vi "RealTimeMain.vi"(9 "For Reference (frames)":i32=1 min=1, 11 "Motion Data":T2(array[cluster])) -> (3 "Array":dbl[][](array[numeric]))   [LabVIEW 2014]
uses:
  GlobalVars.vi
panel:
  out "Averaging 2":bool
  in  "Col Shift Element":dbl[](array[numeric])
  in  "Vert SF":dbl[](array[numeric])
  in  "Row Shift Element":dbl[](array[numeric])
  in  "Horiz SF":dbl[](array[numeric])
  in  "Reference Frame":dbl[][][](array[numeric])
  in  "Header":T1
  in  "Ref Avg Count":i32
  in  "Alarm Structure":enum32{"Alarm", "Averaging"}(tab)=enum."Averaging"
  in  "Averaging":bool
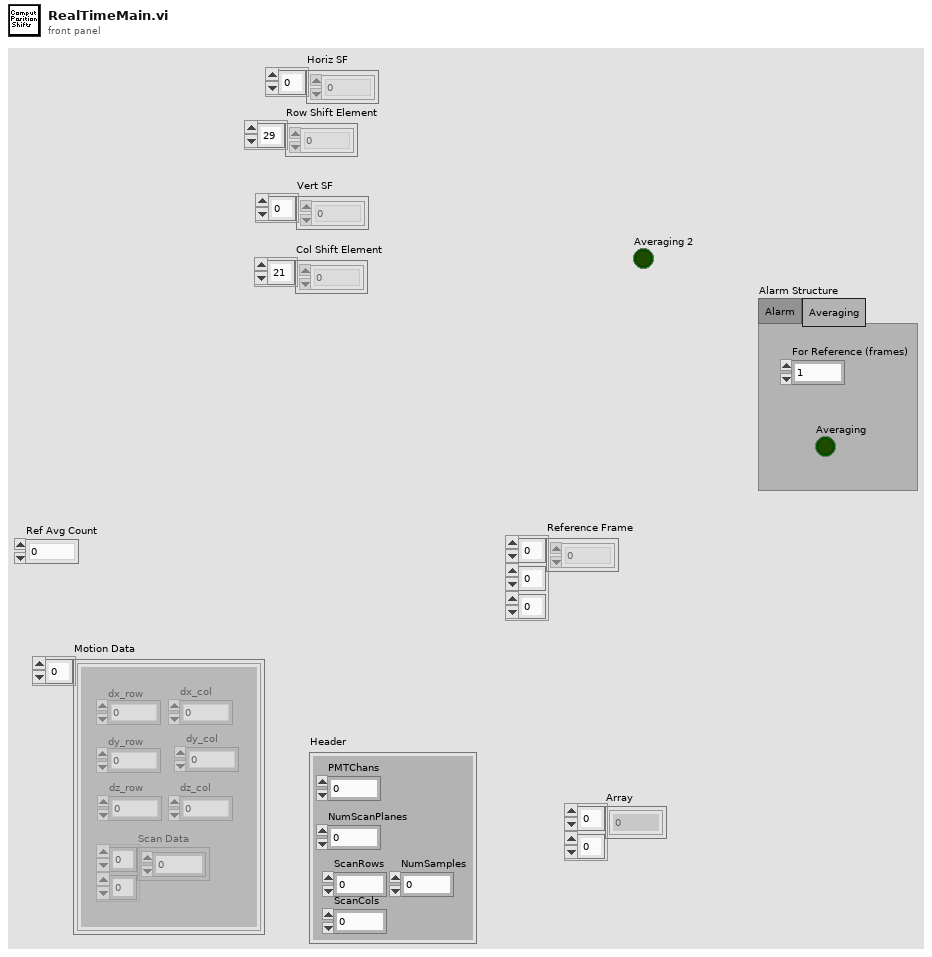
[diagram p1: front panel]
types:
  T1 = cluster{"PMTChans":i32, "NumScanPlanes":i32, "ScanRows":i32, "ScanCols":i32, "NumSamples":i32}
  T2 = cluster{"Scan Data":i32[][], "dx_row":dbl, "dy_row":dbl, "dz_row":dbl, "dx_col":dbl, "dy_col":dbl, "dz_col":dbl}[]
  T3 = cluster{"Scan Data":i32[][], "dx_row":dbl, "dy_row":dbl, "dz_row":dbl, "dx_col":dbl, "dy_col":dbl, "dz_col":dbl}
  T4 = cluster{"dx_row":dbl, "dy_row":dbl, "dz_row":dbl, "dx_col":dbl, "dy_col":dbl, "dz_col":dbl}
  T5 = cluster{"X1":dbl[], "Y1":dbl[], "Z1":dbl[], "X2":dbl[], "Y2":dbl[], "Z2":dbl[]}
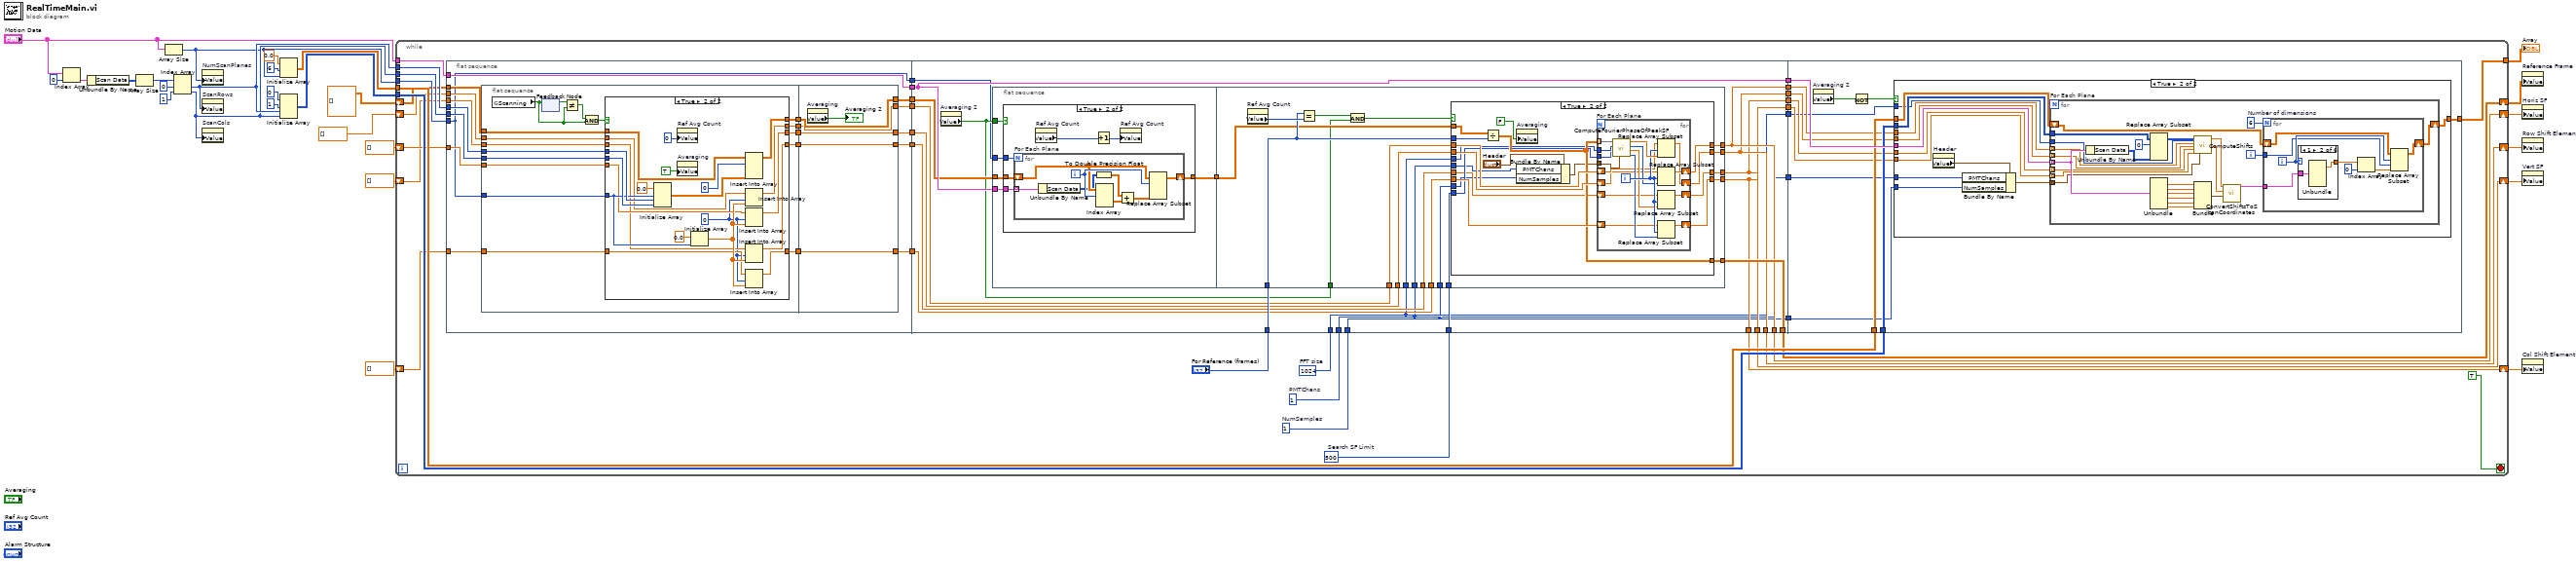
[diagram p0: block diagram]
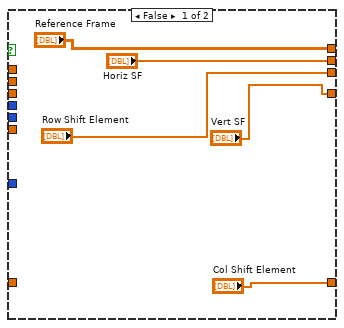
[diagram p2: hidden frame]
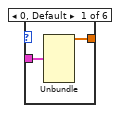
[diagram p6: hidden frame]
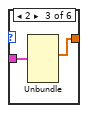
[diagram p7: hidden frame]
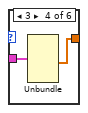
[diagram p8: hidden frame]
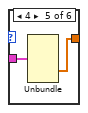
[diagram p9: hidden frame]
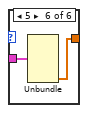
[diagram p10: hidden frame]
diagram:
  n1 = Index Array(array="Motion Data", index=0) -> (element=w26:T3)
  n2 = Unbundle By Name(w26) -> ("Scan Data"=w25:i32[][])
  n3 = Array Size(array=w25) -> (size(s)=w24:i32[])
  n4 = Array Size(array="Motion Data") -> (size(s)=w14:i32)
  n5 = Index Array(array=w24, index #1=0 ("index"), index #2=1 ("index")) -> (element #1=w17:i32, element #2=w16:i32)
  n6 = property on="NumScanPlanes" class="DigNum (strict)"("Value"=w14) -> ()  [unwired: 2 in, 2 out]
  n7 = property on="ScanRows" class="DigNum (strict)"("Value"=w17) -> ()  [unwired: 2 in, 2 out]
  n8 = property on="ScanCols" class="DigNum (strict)"("Value"=w16) -> ()  [unwired: 2 in, 2 out]
  n9 = Initialize Array(0.0 ("element"), 6 ("dimension size"), w14) -> (w12:dbl[][])
  n10 = Initialize Array(0 ("element"), 1 ("dimension size"), w17, w16) -> (w18:i32[][][])
  n11 = while {
    tunnel: "Motion Data" -> [w54]
    tunnel: w18 -> [w52]
    tunnel: w17 -> [w51]
    tunnel: w16 -> [w50]
    tunnel: w14 -> [w49]
    tunnel: w12 -> [w48]
    shift-right: [w42] -> w11
    shift-left: dbl[][][] [] -> [w35]
    tunnel: [w43] -> w6
    shift-right: [w41] -> w10
    shift-left: dbl[] [] -> [w47]
    shift-right: [w40] -> w9
    shift-left: dbl[] [] -> [w46]
    shift-right: [w39] -> w8
    shift-left: dbl[] [] -> [w45]
    shift-right: [w38] -> w7
    shift-left: dbl[] [] -> [w44]
    stop <- TRUE stop-if-true
    w30 = 1  # NumSamples
    w31 = 1  # PMTChans
    w34 = 500  # Search SF Limit
    w33 = 1024  # FFT size
    n12 = flat-sequence {
      tunnel: w54 -> [w84]
      tunnel: [w84] -> w65
      tunnel: w49 -> [w66]
      tunnel: w51 -> [w83]
      tunnel: w50 -> [w67]
      tunnel: w35 -> [w82]
      tunnel: [w81] -> w64
      tunnel: w47 -> [w80]
      tunnel: w46 -> [w79]
      tunnel: w45 -> [w78]
      tunnel: w44 -> [w77]
      tunnel: [w76] -> w63
      tunnel: [w75] -> w62
      tunnel: [w74] -> w61
      tunnel: [w73] -> w60
      tunnel: [w66] -> w37
      tunnel: w65 -> [w150]
      tunnel: "For Reference (frames)" -> [w152]
      tunnel: [w150] -> w59
      tunnel: w64 -> [w149]
      tunnel: w63 -> [w148]
      tunnel: w62 -> [w147]
      tunnel: w61 -> [w146]
      tunnel: w60 -> [w145]
      tunnel: [w142] -> w58
      tunnel: [w141] -> w57
      tunnel: [w140] -> w56
      tunnel: [w139] -> w55
      tunnel: [w143] -> w42
      tunnel: [w142] -> w41
      tunnel: [w141] -> w40
      tunnel: [w140] -> w39
      tunnel: [w139] -> w38
      tunnel: w37 -> [w138]
      tunnel: w33 -> [w136]
      tunnel: w34 -> [w137]
      tunnel: [w136] -> w32
      tunnel: w31 -> [w134]
      tunnel: w30 -> [w135]
      tunnel: [w135] -> w29
      tunnel: [w134] -> w28
      tunnel: w59 -> [w244]
      tunnel: w52 -> [w243]
      tunnel: w48 -> [w242]
      tunnel: w58 -> [w241]
      tunnel: w57 -> [w240]
      tunnel: w56 -> [w239]
      tunnel: w55 -> [w238]
      tunnel: [w237] -> w43
      tunnel: w32 -> [w234]
      tunnel: w29 -> [w233]
      tunnel: w28 -> [w232]
      frame #0 {
        n13 = flat-sequence {
          tunnel: w66 -> [w101]
          tunnel: w83 -> [w100]
          tunnel: w67 -> [w99]
          tunnel: w82 -> [w98]
          tunnel: w80 -> [w96]
          tunnel: w79 -> [w95]
          tunnel: w78 -> [w94]
          tunnel: w77 -> [w93]
          tunnel: [w97] -> w72
          tunnel: [w92] -> w71
          tunnel: [w91] -> w70
          tunnel: [w90] -> w69
          tunnel: [w89] -> w68
          tunnel: [w129] -> w73
          tunnel: [w130] -> w74
          tunnel: [w131] -> w75
          tunnel: [w132] -> w76
          tunnel: [w133] -> w81
          tunnel: w72 -> [w133]
          tunnel: w71 -> [w132]
          tunnel: w70 -> [w131]
          tunnel: w69 -> [w130]
          tunnel: w68 -> [w129]
          frame #0 {
            n14 = global read "GlobalVars.vi" "Scanning"() -> (w86:bool)
            n15 = feedback-in #1(w86) -> ()
            n16 = feedback #1() -> (w88:bool)  [unwired: 1 in]
            n17 = Not Equal?(x=w88, y=w86) -> (x != y?=w87:bool)
            n18 = And(x=w87, y=w86) -> (x .and. y?=w85:bool)
            n19 = case shown="True" w85 {
              tunnel: w101 -> [_ w119]
              tunnel: w100 -> [_ w126]
              tunnel: w99 -> [_ w125]
              tunnel: w98 -> [_ w124]
              tunnel: ["Reference Frame" w122] -> w97
              tunnel: w96 -> [_ w118]
              tunnel: w95 -> [_ w116]
              tunnel: w94 -> [_ w115]
              tunnel: w93 -> [_ w114]
              tunnel: ["Horiz SF" w112] -> w92
              tunnel: ["Row Shift Element" w111] -> w91
              tunnel: ["Vert SF" w110] -> w90
              tunnel: ["Col Shift Element" w109] -> w89
              frame False {
              }
              frame True {
                w107 = 0 ("index")
                n20 = Initialize Array(0.0 ("element"), w119, w126, w125) -> (w123:dbl[][][])
                n21 = property on="Ref Avg Count" class="DigNum (strict)"("Value"=0 ("Ref Avg Count")) -> ()  [unwired: 2 in, 2 out]
                n22 = property on="Averaging" class="Bool (strict)"("Value"=TRUE) -> ()  [unwired: 2 in, 2 out]
                n23 = Initialize Array(0.0 ("element"), w119) -> (w117:dbl[])
                n24 = Insert Into Array(array=w124, index (dim 0)=0 ("index (page)"), new element=w123) -> (w122:dbl[][][])  [unwired: 2 in]
                n25 = Insert Into Array(array=w118, index=w107, new element=w117) -> (w112:dbl[])
                n26 = Insert Into Array(array=w116, index=w107, new element=w117) -> (w111:dbl[])
                n27 = Insert Into Array(array=w115, index=w107, new element=w117) -> (w110:dbl[])
                n28 = Insert Into Array(array=w114, index=w107, new element=w117) -> (w109:dbl[])
              }
            }
          }
          frame #1 {
            n29 = property on="Averaging" class="Bool (strict)"() -> ("Value"=→"Averaging 2":bool)  [unwired: 2 in, 2 out]
          }
        }
      }
      frame #1 {
        n30 = property on="Averaging 2" class="Bool (strict)"() -> ("Value"=w144:bool)  [unwired: 2 in, 2 out]
        n31 = flat-sequence {
          tunnel: w150 -> [w157]
          tunnel: w144 -> [w156]
          tunnel: [w155] -> w151
          tunnel: w149 -> [w154]
          tunnel: w138 -> [w153]
          tunnel: w152 -> [w188]
          tunnel: w151 -> [w187]
          tunnel: w148 -> [w186]
          tunnel: w147 -> [w185]
          tunnel: w146 -> [w184]
          tunnel: w145 -> [w183]
          tunnel: [w182] -> w142
          tunnel: [w181] -> w141
          tunnel: [w180] -> w140
          tunnel: [w179] -> w139
          tunnel: w144 -> [w178]
          tunnel: [w177] -> w143
          tunnel: w136 -> [w176]
          tunnel: w137 -> [w175]
          tunnel: w134 -> [w174]
          tunnel: w135 -> [w173]
          frame #0 {
            n32 = case shown="True" w156 {
              tunnel: w157 -> [_ w164]
              tunnel: [w158 w163] -> w155
              tunnel: w154 -> [w158 w162]
              tunnel: w153 -> [_ w159]
              frame False {
              }
              frame True {
                n33 = for "For Each Plane" {
                  N: w159 -> [_]
                  tunnel: w164 -> [w172] mode=indexing
                  shift-right: [w167] -> w163
                  shift-left: w162 -> [w169]
                  i -> [w170]
                  n34 = Unbundle By Name(w172) -> ("Scan Data"=w166:i32[][])
                  n35 = To Double Precision Float(number=w166) -> (double precision float=w165:dbl[][])
                  n36 = Index Array(array=w169, index (dim 0)=w170) -> (element=w171:dbl[][])  [unwired: 2 in]
                  n37 = Add(x=w165, y=w171) -> (x+y=w168:dbl[][])
                  n38 = Replace Array Subset(array=w169, new element=w168, index (dim 0)=w170) -> (w167:dbl[][][])  [unwired: 2 in]
                }
                n39 = property on="Ref Avg Count" class="DigNum (strict)"() -> ("Value"=w161:i32)  [unwired: 2 in, 2 out]
                n40 = Increment(x=w161) -> (x+1=w160:i32)
                n41 = property on="Ref Avg Count" class="DigNum (strict)"("Value"=w160) -> ()  [unwired: 2 in, 2 out]
              }
            }
          }
          frame #1 {
            n42 = property on="Ref Avg Count" class="DigNum (strict)"() -> ("Value"=w189:i32)  [unwired: 2 in, 2 out]
            n43 = Equal?(x=w188, y=w189) -> (x = y?=w191:bool)
            n44 = And(x=w191, y=w178) -> (x .and. y?=w190:bool)
            n45 = case shown="True" w190 {
              tunnel: w187 -> [w192 w214]
              tunnel: w188 -> [_ w213]
              tunnel: w186 -> [w193 w212]
              tunnel: w185 -> [w194 w211]
              tunnel: w184 -> [w195 w198]
              tunnel: w183 -> [w196 w210]
              tunnel: [w193 w209] -> w182
              tunnel: [w194 w208] -> w181
              tunnel: [w195 w207] -> w180
              tunnel: [w196 w206] -> w179
              tunnel: [w192 w204] -> w177
              tunnel: w176 -> [_ w201]
              tunnel: w175 -> [_ w200]
              tunnel: w174 -> [_ w199]
              tunnel: w173 -> [_ w197]
              frame False {
              }
              frame True {
                n46 = Divide(x=w214, y=w213) -> (x/y=w204:dbl[][][])
                n47 = property on="Averaging" class="Bool (strict)"("Value"=FALSE) -> ()  [unwired: 2 in, 2 out]
                n48 = Bundle By Name(cluster="Header", "PMTChans"=w199, "NumSamples"=w197) -> (w202:T1)
                n49 = for "For Each Plane" {
                  tunnel: w204 -> [w231] mode=indexing
                  shift-right: [w221] -> w209
                  shift-left: w212 -> [w225]
                  shift-right: [w220] -> w208
                  shift-left: w211 -> [w224]
                  shift-right: [w219] -> w207
                  shift-left: w198 -> [w223]
                  shift-right: [w218] -> w206
                  shift-left: w210 -> [w222]
                  tunnel: w202 -> [w217]
                  tunnel: w201 -> [w216]
                  tunnel: w200 -> [w215]
                  i -> [w229]
                  n50 = call "ComputeFourierPhaseOfPeakSF.vi"("Header"=w217, "Search SF Limit"=w215, "FFT size"=w216, "Scan Frame"=w231) -> ("Col Shift Element Number"=w226:i32, "Vertical SF Phase"=w227:dbl, "Row Shift Element Numbert"=w228:i32, "Horizontal SF Phase"=w230:dbl)  [unwired: 4 in]
                  n51 = Replace Array Subset(array=w225, new element=w230, index=w229) -> (w221:dbl[])
                  n52 = Replace Array Subset(array=w224, new element=w228, index=w229) -> (w220:dbl[])
                  n53 = Replace Array Subset(array=w223, new element=w227, index=w229) -> (w219:dbl[])
                  n54 = Replace Array Subset(array=w222, new element=w226, index=w229) -> (w218:dbl[])
                }
              }
            }
          }
        }
      }
      frame #2 {
        n55 = property on="Averaging 2" class="Bool (strict)"() -> ("Value"=w236:bool)  [unwired: 2 in, 2 out]
        n56 = Not(x=w236) -> (.not. x?=w235:bool)
        n57 = case shown="True" w235 {
          tunnel: w244 -> [_ w258]
          tunnel: w243 -> [_ w257]
          tunnel: [w245 w256] -> w237
          tunnel: w242 -> [w245 w255]
          tunnel: w241 -> [_ w254]
          tunnel: w240 -> [_ w253]
          tunnel: w239 -> [_ w252]
          tunnel: w238 -> [_ w251]
          tunnel: w234 -> [_ w248]
          tunnel: w233 -> [_ w247]
          tunnel: w232 -> [_ w246]
          frame False {
          }
          frame True {
            n58 = property on="Header" class="Clust (strict)"() -> ("Value"=w250:T1)  [unwired: 2 in, 2 out]
            n59 = Bundle By Name(cluster=w250, "PMTChans"=w246, "NumSamples"=w247) -> (w249:T1)
            n60 = for "For Each Plane" {
              tunnel: w258 -> [w277] mode=indexing
              tunnel: w257 -> [w281]
              tunnel: w249 -> [w270]
              shift-right: [w268] -> w256
              shift-left: w255 -> [w269]
              tunnel: w254 -> [w264] mode=indexing
              tunnel: w253 -> [w263] mode=indexing
              tunnel: w252 -> [w262] mode=indexing
              tunnel: w251 -> [w261] mode=indexing
              tunnel: w248 -> [w260]
              i -> [w267]
              w265 = 6  # Number of dimensions
              n61 = Unbundle By Name(w277) -> ("Scan Data"=w279:i32[][])
              n62 = Replace Array Subset(array=w281, new element=w279, index (dim 0)=0 ("index (row)")) -> (w278:i32[][][])  [unwired: 2 in]
              n63 = Unbundle(w277) -> ("dx_row"=w276:dbl, "dy_row"=w275:dbl, "dz_row"=w274:dbl, "dx_col"=w273:dbl, "dy_col"=w272:dbl, "dz_col"=w271:dbl)  [unwired: 1 out]
              n64 = call "ComputeShifts.vi"("Scan Plane Data"=w278, "FFT size"=w260, "Ref Horizontal SF Phase"=w264, "Ref Row Shift Element"=w263, "Ref Vertical SF Phase"=w262, "Ref Col Shift Element"=w261, "Header"=w270) -> ("Row Shift Array"=w283:dbl[], "Col Shift Array"=w282:dbl[])  [unwired: 11 in]
              n65 = Bundle("dx_row"=w276, "dy_row"=w275, "dz_row"=w274, "dx_col"=w273, "dy_col"=w272, "dz_col"=w271) -> (w259:T4)  [unwired: 1 in]
              n66 = call "ConvertShiftsToScanCoordinates.vi"("PixelToScanCoordConvFactors"=w259, "Col Shift Array"=w282, "Row Shift Array"=w283) -> ("Motion"=w266:T5)  [unwired: 8 in]
              n67 = for {
                N: w265 -> [_]
                shift-right: [w284] -> w268
                shift-left: w269 -> [w287]
                tunnel: w267 -> [w285]
                tunnel: w266 -> [w291]
                i -> [w286]
                n68 = case shown="1" w286 {
                  tunnel: [w292 w294 w296 w298 w300 w302] -> w290
                  tunnel: w291 -> [w293 w295 w297 w299 w301 w303]
                  frame 0, Default {
                    n69 = Unbundle(w293) -> ("X1"=w292:dbl[])  [unwired: 5 out]
                  }
                  frame 1 {
                    n70 = Unbundle(w295) -> ("Y1"=w294:dbl[])  [unwired: 5 out]
                  }
                  frame 2 {
                    n71 = Unbundle(w297) -> ("Z1"=w296:dbl[])  [unwired: 5 out]
                  }
                  frame 3 {
                    n72 = Unbundle(w299) -> ("X2"=w298:dbl[])  [unwired: 5 out]
                  }
                  frame 4 {
                    n73 = Unbundle(w301) -> ("Y2"=w300:dbl[])  [unwired: 5 out]
                  }
                  frame 5 {
                    n74 = Unbundle(w303) -> ("Z2"=w302:dbl[])  [unwired: 5 out]
                  }
                }
                n75 = Index Array(array=w290, index=0) -> (element=w288:dbl)
                n76 = Replace Array Subset(array=w287, new element=w288, index (row)=w286, index (col)=w285) -> (w284:dbl[][])
              }
            }
          }
        }
      }
    }
  }
  "Array" <- w6
  n77 = property on="Reference Frame" class="Arr (strict)"("Value"=w11) -> ()  [unwired: 2 in, 2 out]
  n78 = property on="Horiz SF" class="Arr (strict)"("Value"=w10) -> ()  [unwired: 2 in, 2 out]
  n79 = property on="Row Shift Element" class="Arr (strict)"("Value"=w9) -> ()  [unwired: 2 in, 2 out]
  n80 = property on="Vert SF" class="Arr (strict)"("Value"=w8) -> ()  [unwired: 2 in, 2 out]
  n81 = property on="Col Shift Element" class="Arr (strict)"("Value"=w7) -> ()  [unwired: 2 in, 2 out]
